vi "prueba2.vi"(7 "module path":path=path "C:/Users/Taboada.r248/Documents/LabVIEW Projects/LabVIEW-2024-and-Python/pyhthon_modules/find_consecutive_close_values.py", 9 "tolerance":dbl=4.0 format="%#_13g", 10 "min_threshold":dbl=5.0 format="%#_13g", 11 "data":dbl[](array[numeric])) -> (1 "num_elements_found":i32, 2 "data qty":i32, 3 "Measures":dbl[][](array[numeric]), 4 "close_values":dbl[](array[numeric]) format="%.2f", 5 "average":dbl)   [LabVIEW 2024]
panel:
  in  "data 2":dbl[](array[numeric])=[6.606, 6.606, 6.589, 6.623, 6.597, 6.581, 6.542, 24.697, 42.944, 59.771, 76.679, 93.739, 92.297, 90.852, 90.746, 83.923, 76.869, 69.696, 61.389, 52.616, 50.01, 47.013, 44.417, 42.793, 41.744, 44.685, 48.094, 51.47, 54.919, 58.381, 58.325, 58.256, 58.399, 58.525, 58.66, 57.545, 56.393, 55.106, 53.011, 51.038, 50.361, 49.681, 48.971, 49.107, 49.241, 49.229, 49.242, 49.358, 49.366, 49.424]
  out "Measures Plot":dbl[][](graph)
  out "close_values_w_zeros":dbl[](array[numeric]) format="%.2f"
  in  "data1":dbl[](array[numeric])=[0.0, 0.0, 1.0, 2.0, 3.0, 9.3, 9.4, 9.5, 9.4, 9.2, 9.1, 5.0, 4.5, 4.0, 3.0, 2.0, 1.0, 0.0, 0.0] format="%.2f"
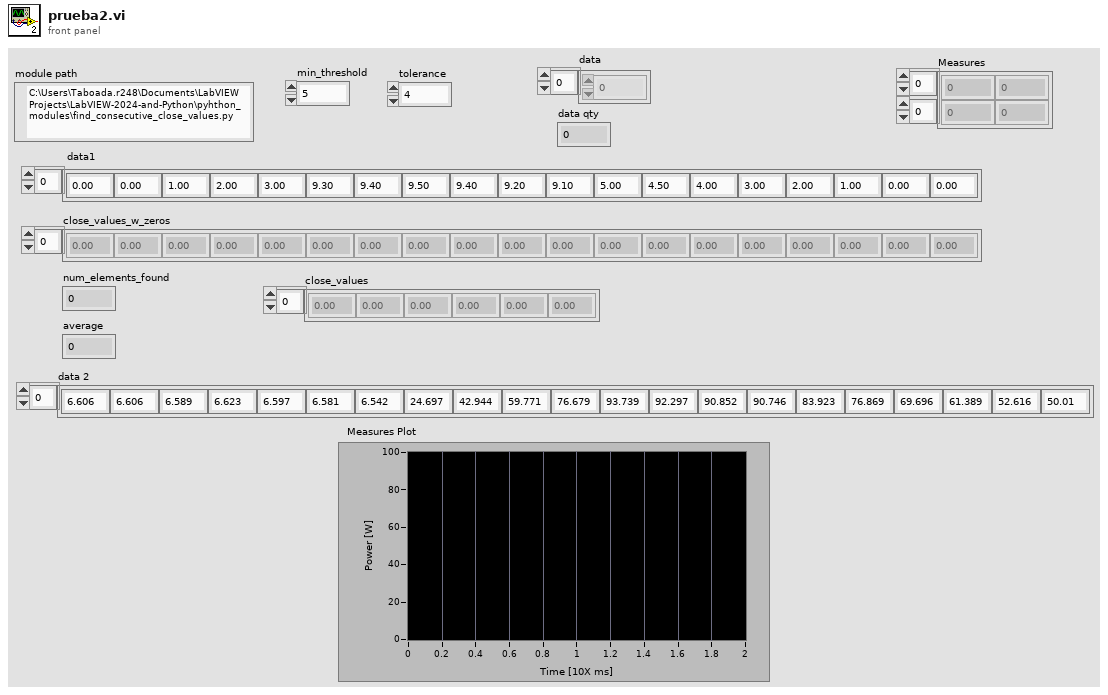
[diagram p1: front panel]
types:
  T1 = cluster{"close_values_w_zeros":dbl[], "num_elements_found":i32, "close_values":dbl[], "average":dbl}
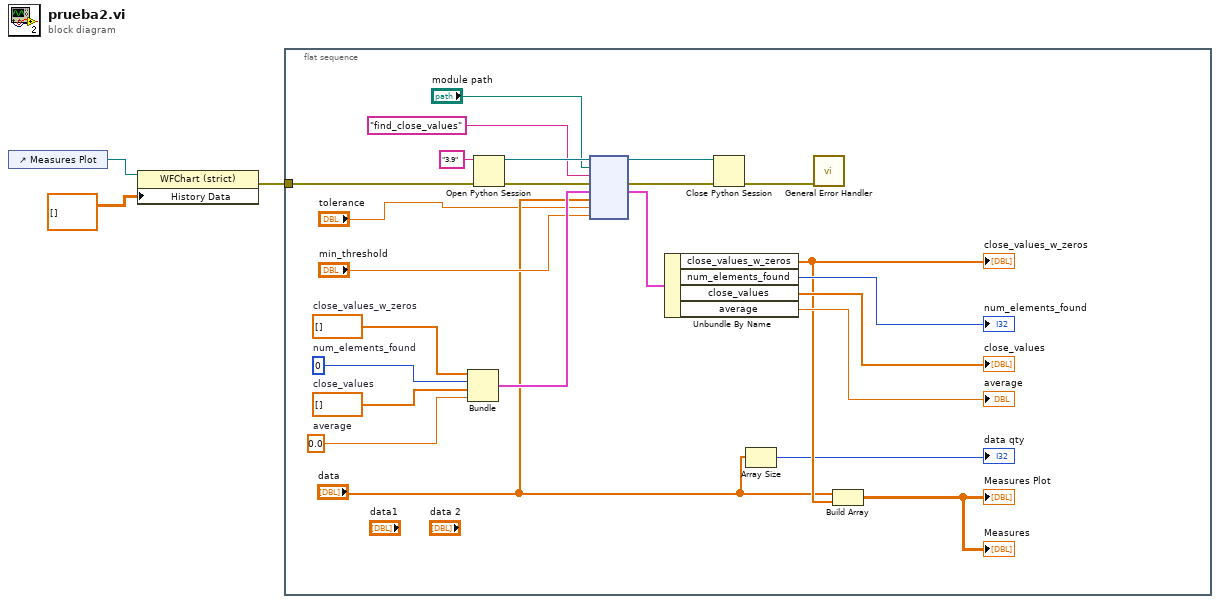
[diagram p0: block diagram]
diagram:
  n1 = control-ref of="Measures Plot"() -> (w3:refnum<vi>)
  n2 = property class="WFChart (strict)"(reference=w3, "History Data"=dbl[][] []) -> (error out=w1:errorcluster)  [unwired: 1 in, 1 out]
  n3 = flat-sequence {
    tunnel: w1 -> [w9]
    frame #0 {
      w16 = 0.0  # average
      w17 = dbl[] []  # close_values
      w18 = 0  # num_elements_found
      w19 = dbl[] []  # close_values_w_zeros
      n4 = Bundle("close_values_w_zeros"=w19, "num_elements_found"=w18, "close_values"=w17, "average"=w16) -> (w15:T1)  [unwired: 1 in]
      n5 = Open Python Session(python version="3.9" ("Python version"), 3:w9) -> (session out=w24:refnum<k35>, error out=w27:errorcluster)  [unwired: 1 in]
      n6 = node(w24, "module path", "find_close_values" ("function name"), w27, w15, "data", "tolerance", "min_threshold") -> (w23:refnum<k35>, w26:errorcluster, w13:T1)  [unwired: 3 in, 2 out]
      n7 = Unbundle By Name(w13) -> ("close_values_w_zeros"=w8:dbl[], "num_elements_found"=→"num_elements_found":i32, "close_values"=→"close_values":dbl[], "average"=→"average":dbl)
      "close_values_w_zeros" <- w8
      n8 = Close Python Session(session in=w23, error in=w26) -> (11:w22:errorcluster)
      n9 = Array Size(array="data") -> (size(s)=→"data qty":i32)
      n10 = call <vilib>:"General Error Handler.vi"("error in (no error)"=w22) -> ()  [unwired: 10 in, 5 out]
      n11 = Build Array("data", w8) -> (→"Measures Plot" →"Measures":dbl[][])
    }
  }
